vi "MAT_Header.vi"(11 "Title String":string="MATLAB 5.0 MAT-file, Platform: MACI64, Created on: Mon Sep 14 17:22:31 2015                                         ") -> (3 "String out":string)   [LabVIEW 2022 SP3]
panel:
  out "Check?":bool
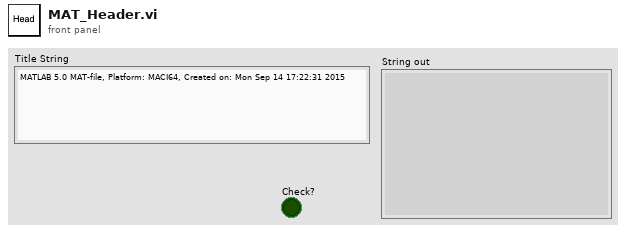
[diagram p1: front panel]
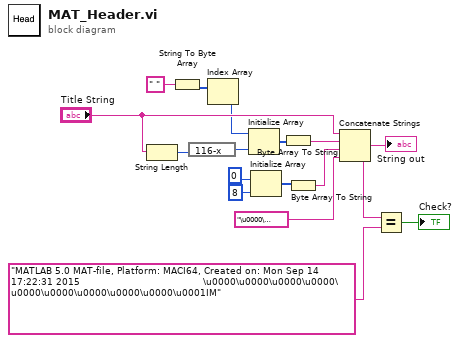
[diagram p0: block diagram]
diagram:
  n1 = String Length(string="Title String") -> (length=w7:i32)
  n2 = String To Byte Array(string=" ") -> (unsigned byte array=w2:u8[])
  n3 = expression code="116-x"(w7) -> (w8:i32)
  n4 = Index Array(array=w2) -> (element=w1:u8)  [unwired: 1 in]
  n5 = Initialize Array(w1, w8) -> (w9:u8[])
  n6 = Initialize Array(u8 0 ("element"), 8 ("dimension size")) -> (w13:u8[])
  n7 = Byte Array To String(unsigned byte array=w9) -> (string=w10:string)
  n8 = Byte Array To String(unsigned byte array=w13) -> (string=w14:string)
  n9 = Concatenate Strings("Title String", w10, w14, "\u0000\u0001IM" ("substring before match")) -> (w6:string)
  "String out" <- w6
  n10 = Equal?(x=w6, y="MATLAB 5.0 MAT-file, Platform: MACI64, Created on: Mon Sep 14 17:22:31 2015                                         \u0000\u0000\u0000\u0000\u0000\u0000\u0000\u0000\u0000\u0001IM" ("data")) -> (x = y?=→"Check?":bool)
